vi "SE FP hindbrain SENSE.vi"(0 "Old X Position":i32, 1 "Old Y Position":i32, 3 "GPS":cluster{"X pos":i32, "Y pos":i32, "Heading":dbl}, 5 "IR Sensors":T1(array[cluster]), 7 "Old Speed of Boat\nin Pixels/Sec":dbl, 9 "Analog Input Values":dbl[](array[numeric]), 11 "error in":errorcluster) -> (4 "Boat Status":T2, 6 "IR Sensors 2":T1(array[cluster]), 10 "error out":errorcluster, 12 "New X Position":i32, 14 "New Speed of Boat\nin Pixels/Sec":dbl, 15 "New Y Position":i32)   [LabVIEW 2014]
doc: "This vi calculate the distance from the boat edge to the detected object. If no object is detected the value is 0. It also determines of the boat is out of power...if so it will stop the boat."
panel:
  out "RIO BAT":dbl
  out "MOT BAT":dbl
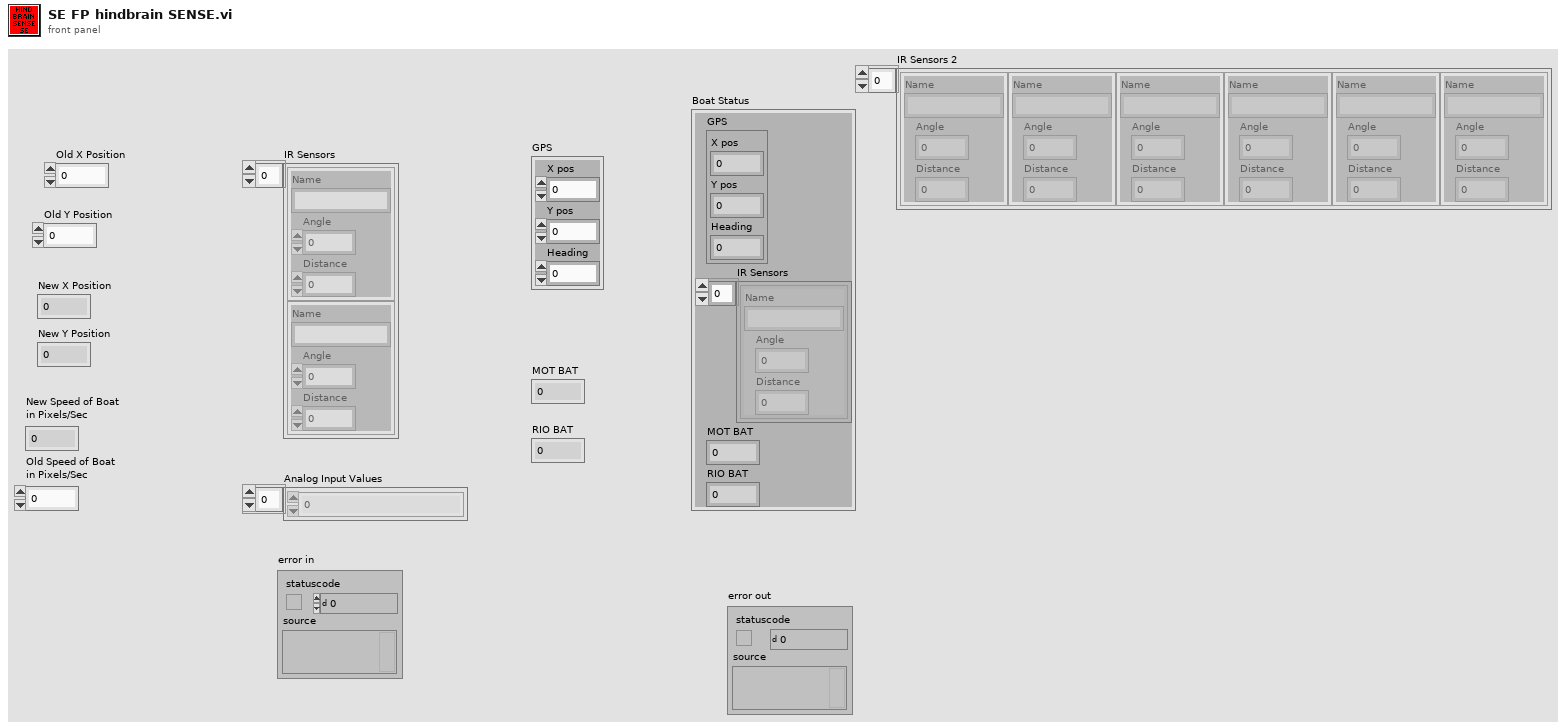
[diagram p1: front panel]
types:
  T1 = cluster{"Name":string, "Angle":dbl, "Distance":dbl}[]
  T2 = cluster{"GPS":cluster{"X pos":i32, "Y pos":i32, "Heading":dbl}, "IR Sensors":cluster{"Name":string, "Angle":dbl, "Distance":dbl}[], "MOT BAT":dbl, "RIO BAT":dbl}
  T3 = cluster{"Name":string, "Angle":dbl, "Distance":dbl}
  T4 = cluster{"GPS":cluster{"X pos":i32, "Y pos":i32, "Heading":dbl}, cluster{"Name":string, "Angle":dbl, "Distance":dbl}[], "MOT BAT":dbl, "RIO BAT":dbl}
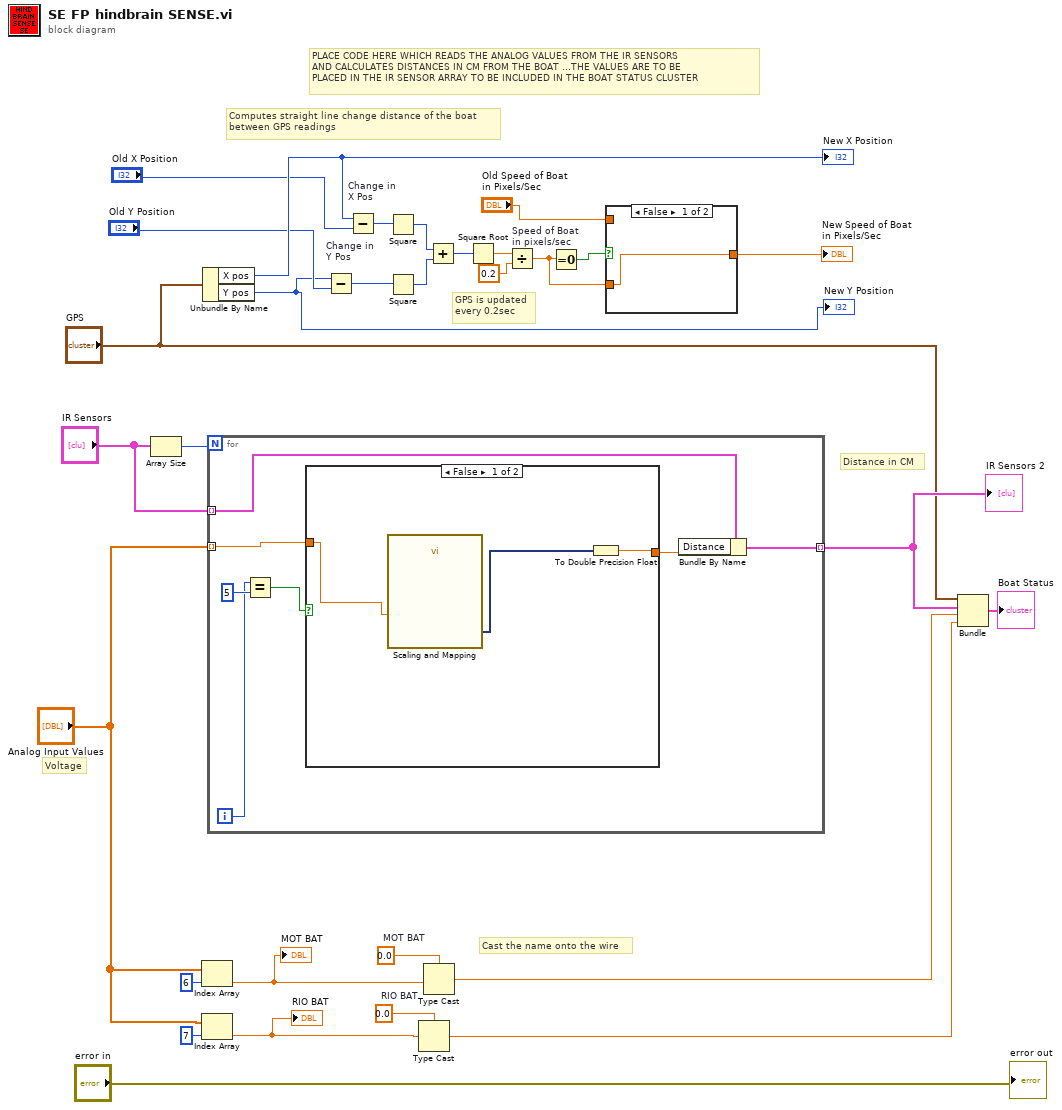
[diagram p0: block diagram]
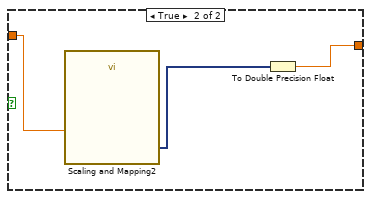
[diagram p3: hidden frame]
diagram:
  w24 = 0.0  # RIO BAT
  w28 = 0.0  # MOT BAT
  # "GPS is updated\nevery 0.2sec"
  # "Computes straight line change distance of the boat\nbetween GPS readings"
  # "Voltage"
  # "Distance in CM"
  # "PLACE CODE HERE WHICH READS THE ANALOG VALUES FROM THE IR SENSORS \nAND CALCULATES DISTANCES IN CM FROM THE BOAT ...THE VALUES ARE TO BE \nPLACED IN THE IR SENSOR ARRAY TO BE INCLUDED IN THE BOAT STATUS CLUSTER"
  # "Cast the name onto the wire"
  n1 = Array Size(array="IR Sensors") -> (size(s)=w19:i32)
  n2 = Index Array(array="Analog Input Values", index=6) -> (element=w27:dbl)
  "MOT BAT" <- w27
  n3 = Index Array(array="Analog Input Values", index=7) -> (element=w23:dbl)
  "RIO BAT" <- w23
  n4 = Unbundle By Name("GPS") -> ("X pos"=w15:i32, "Y pos"=w5:i32)
  "New X Position" <- w15
  "New Y Position" <- w5
  n5 = for {
    N: w19 -> [_]
    tunnel: "IR Sensors" -> [w35] mode=indexing
    tunnel: "Analog Input Values" -> [w34] mode=indexing
    tunnel: [w37] -> w18 mode=indexing
    i -> [w31]
    n6 = Equal?(x=w31, y=5) -> (x = y?=w33:bool)
    n7 = case shown="False" w33 {
      tunnel: [w40 w43] -> w36
      tunnel: w34 -> [w39 w41]
      frame False {
        n8 = call "Scaling and Mapping"("Signals"=w39) -> ("Scaled Signals"=w38:dynamicdata)  [unwired: 9 in, 1 out]
        n9 = To Double Precision Float(number=w38) -> (double precision float=w40:dbl)
      }
      frame True {
        n10 = call "Scaling and Mapping2"("Signals"=w41) -> ("Scaled Signals"=w42:dynamicdata)  [unwired: 9 in, 1 out]
        n11 = To Double Precision Float(number=w42) -> (double precision float=w43:dbl)
      }
    }
    n12 = Bundle By Name(cluster=w35, "Distance"=w36) -> (w37:T3)
  }
  "IR Sensors 2" <- w18
  n13 = Subtract "Change in \nY Pos"(x=w5, y="Old Y Position") -> (x-y=w13:i32)
  n14 = Subtract "Change in \nX Pos"(x=w15, y="Old X Position") -> (x-y=w14:i32)
  n15 = Square(x=w14) -> (x^2=w11:i32)
  n16 = Square(x=w13) -> (x^2=w12:i32)
  n17 = Type Cast(type=w24, x=w23) -> (*(type *) &x=w22:dbl)
  n18 = Type Cast(type=w28, x=w27) -> (*(type *) &x=w26:dbl)
  n19 = Add(x=w11, y=w12) -> (x+y=w10:i32)
  n20 = Square Root(x=w10) -> (sqrt(x)=w7:dbl)
  n21 = Divide "Speed of Boat\nin pixels/sec"(x=w7, y=0.2) -> (x/y=w3:dbl)
  n22 = Equal To 0?(x=w3) -> (x = 0?=w4:bool)
  n23 = case shown="False" w4 {
    tunnel: w3 -> [w44 _]
    tunnel: "Old Speed of Boat\nin Pixels/Sec" -> [_ w45]
    tunnel: [w44 w45] -> w1
    frame False {
    }
    frame True {
    }
  }
  "New Speed of Boat\nin Pixels/Sec" <- w1
  n24 = Bundle("GPS"="GPS", w18, "MOT BAT"=w26, "RIO BAT"=w22) -> (→"Boat Status":T4)  [unwired: 1 in]
  "error out" <- "error in"
